vi "task id offset.vi"() -> (0 "taskID offset":i32 format="%.0x")   [LabVIEW 2011]
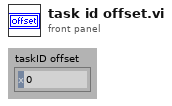
[diagram p1: front panel]
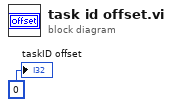
[diagram p0: block diagram]
diagram:
  "taskID offset" <- 0 ("y")
